vi "Type Color.vi"(11 "DoublePanel in":refnum<class "DoublePanel.lvclass">) -> (2 "Type Color":u32(colorbox))   [LabVIEW 2020, in "Conditum-Tools.lvlib" / "DoublePanel.lvclass"]
uses:
  DoublePanel.lvclass
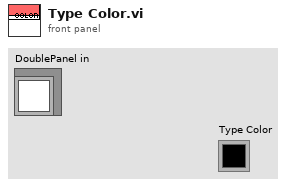
[diagram p1: front panel]
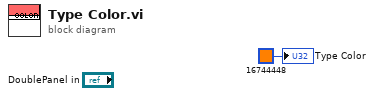
[diagram p0: block diagram]
diagram:
  "Type Color" <- u32 16744448 ("Type Color")
